vi "4155C Output Config SMUs v2.0.vi"(0 "VISA resource name in":refnum<visa-resource-name>, 1 "sweep method":u16(ring) items=["Continuous", "Pulsed"], 2 "Gate mode":u16(ring)=2 items=["Auto", "Limited", "Fixed"], 3 "Gate Range":u8(slide)=2 max=11 scale=0.0..11.0, 5 "Pulse period":dbl=0.005 min=0.005 max=1.0 step=0.0001 format="%.4f", 7 "Pulse width":dbl=0.0005 min=0.0005 max=0.1 step=0.0001 format="%.4f", 8 "Drain Standby":bool, 9 "Base voltage":dbl format="%^.4e", 10 "Gate Standby":bool, 11 "error in (no error)":errorcluster, 12 "SMU4":cluster{"on/off":bool, "Voltage":dbl} {"Voltage" min=-100.0 max=100.0 format="%.2f"}, 13 "Source/drain mode":u16(ring)=2 items=["Auto", "Limited", "Fixed"], 14 "Source/drain Range":u8(slide)=2 max=11 scale=0.0..11.0) -> (4 "VISA Resource Name out":refnum<visa-resource-name>, 15 "error out":errorcluster)   [LabVIEW 2016]
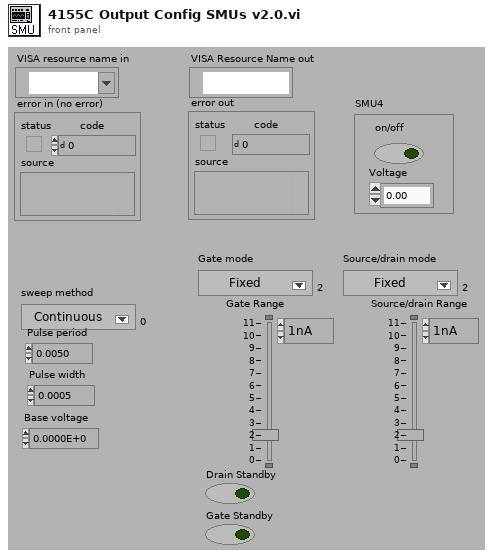
[diagram p1: front panel]
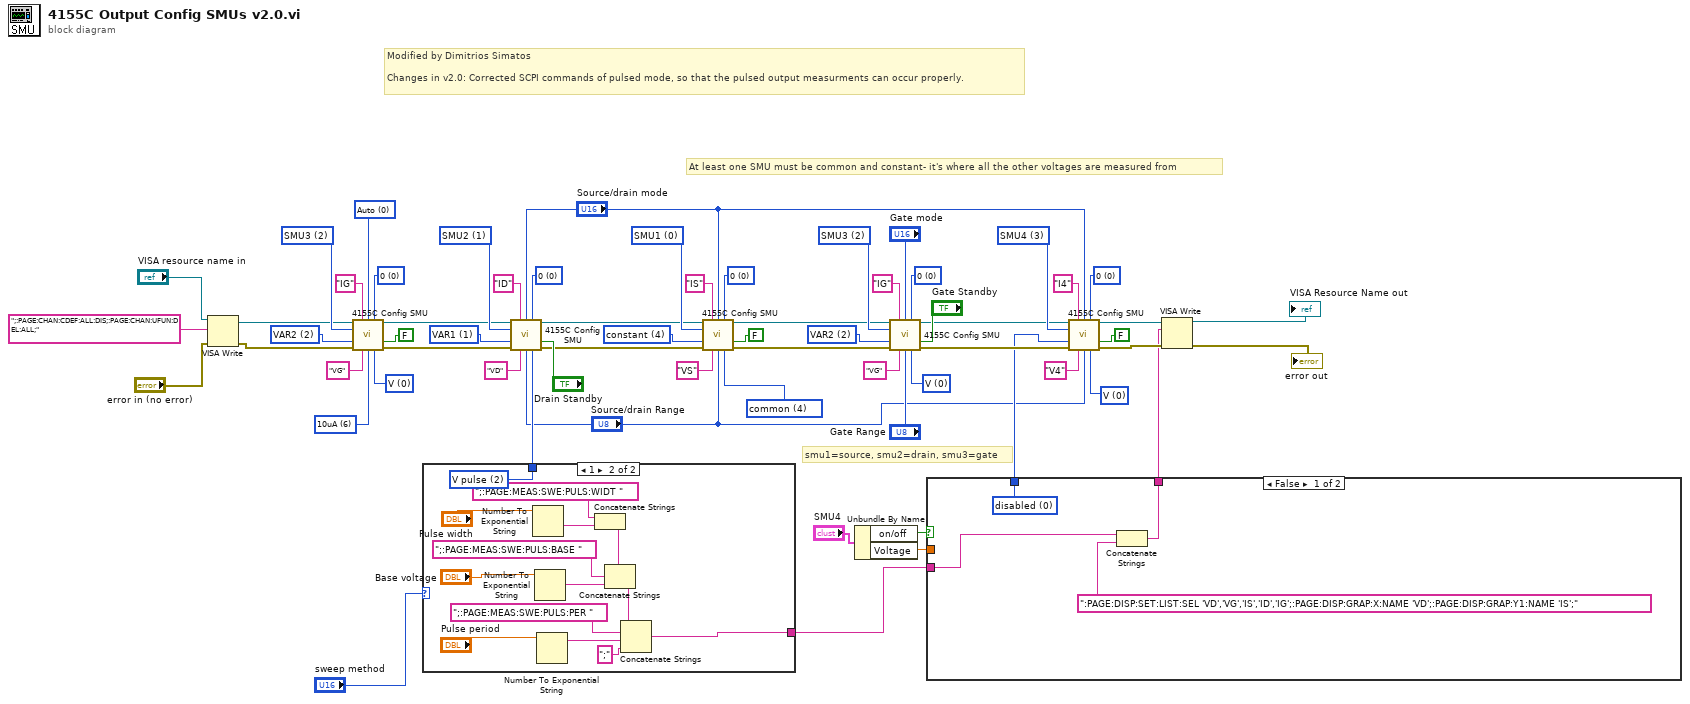
[diagram p0: block diagram]
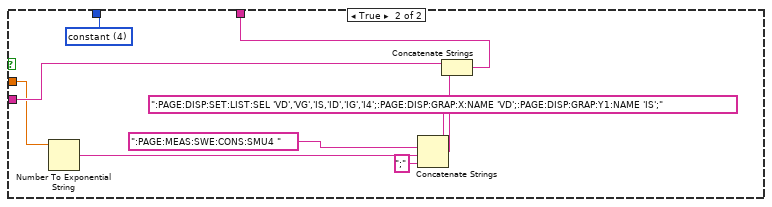
[diagram p2: hidden frame]
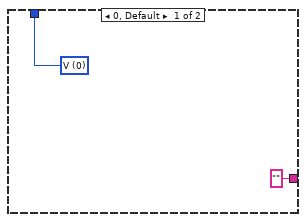
[diagram p3: hidden frame]
diagram:
  w8 = u32 0 items=["V  ", "I  ", "V pulse  ", "I pulse  ", "  common  "] ("mode")
  w15 = u16 0 items=["Auto", "Limited", "Fixed"] ("Range mode")
  w16 = u8 6 items=["10fA  ", "100fA  ", "1nA  ", "10nA", "100nA", "1uA", "10uA", "100uA", "1mA", "10mA", "100mA", "1A"] ("Range")
  w19 = u32 2 items=["SMU1  ", "SMU2  ", "SMU3  ", "SMU4  ", "SMU5  ", "SMU6  "] ("unit to configure")
  w20 = u32 2 items=["disabled  ", "VAR1  ", "VAR2  ", "VAR1'  ", "constant  "] ("function")
  w22 = u32 0 items=["0  ", "10K Ohms  ", "100K Ohms  ", "1M Ohms  "] ("series resistance *")
  w23 = u32 0 items=["V  ", "I  ", "V pulse  ", "I pulse  ", "  common  "] ("mode")
  w43 = u32 0 items=["0  ", "10K Ohms  ", "100K Ohms  ", "1M Ohms  "] ("series resistance *")
  w45 = u32 3 items=["SMU1  ", "SMU2  ", "SMU3  ", "SMU4  ", "SMU5  ", "SMU6  "] ("unit to configure")
  w48 = u32 0 items=["V  ", "I  ", "V pulse  ", "I pulse  ", "  common  "] ("mode")
  w49 = u32 0 items=["0  ", "10K Ohms  ", "100K Ohms  ", "1M Ohms  "] ("series resistance *")
  w51 = u32 2 items=["disabled  ", "VAR1  ", "VAR2  ", "VAR1'  ", "constant  "] ("function")
  w52 = u32 2 items=["SMU1  ", "SMU2  ", "SMU3  ", "SMU4  ", "SMU5  ", "SMU6  "] ("unit to configure")
  w55 = u32 0 items=["0  ", "10K Ohms  ", "100K Ohms  ", "1M Ohms  "] ("series resistance *")
  w57 = u32 4 items=["disabled  ", "VAR1  ", "VAR2  ", "VAR1'  ", "constant  "] ("function")
  w58 = u32 0 items=["SMU1  ", "SMU2  ", "SMU3  ", "SMU4  ", "SMU5  ", "SMU6  "] ("unit to configure")
  w27 = u32 4 items=["V  ", "I  ", "V pulse  ", "I pulse  ", "  common  "] ("mode")
  w61 = u32 0 items=["0  ", "10K Ohms  ", "100K Ohms  ", "1M Ohms  "] ("series resistance *")
  w63 = u32 1 items=["disabled  ", "VAR1  ", "VAR2  ", "VAR1'  ", "constant  "] ("function")
  w64 = u32 1 items=["SMU1  ", "SMU2  ", "SMU3  ", "SMU4  ", "SMU5  ", "SMU6  "] ("unit to configure")
  # "Modified by Dimitrios Simatos\n\nChanges in v2.0: Corrected SCPI commands of pulsed mode, so that the pulsed output measurments can occur properly."
  # "smu1=source, smu2=drain, smu3=gate"
  # "At least one SMU must be common and constant- it's where all the other voltages are measured from"
  n1 = VISA Write(VISA resource name="VISA resource name in", write buffer=";:PAGE:CHAN:CDEF:ALL:DIS;:PAGE:CHAN:UFUN:DEL:ALL;", error in (no error)="error in (no error)") -> (VISA resource name out=w4:refnum<visa-resource-name>, error out=w5:errorcluster)  [unwired: 1 out]
  n2 = call "4155C Config SMU.vi"("VISA session"=w4, "I name (max 6 chars)"="IG", "Range mode"=w15, "series resistance *"=w22, "unit to configure"=w19, "function"=w20, "standby"=FALSE, "error in (no error)"=w5, "V name (max 6 chars)"="VG", "Range"=w16, "mode"=w23) -> ("dup VISA resource name"=w17:refnum<visa-resource-name>, "error out"=w18:errorcluster)  [unwired: 3 in]
  n3 = case shown="1" "sweep method" {
    tunnel: [w66 w80] -> w26
    tunnel: ["" w71] -> w13
    frame 0, Default {
      w66 = u32 0 items=["V  ", "I  ", "V pulse  ", "I pulse  ", "  common  "] ("mode")
    }
    frame 1 {
      w80 = u32 2 items=["V  ", "I  ", "V pulse  ", "I pulse  ", "  common  "] ("mode")
      n4 = Number To Exponential String(number="Pulse width") -> (E-format string=w79:string)  [unwired: 3 in]
      n5 = Number To Exponential String(number="Base voltage") -> (E-format string=w75:string)  [unwired: 3 in]
      n6 = Number To Exponential String(number="Pulse period") -> (E-format string=w72:string)  [unwired: 3 in]
      n7 = Concatenate Strings(";:PAGE:MEAS:SWE:PULS:WIDT " ("Substring"), w79) -> (w77:string)
      n8 = Concatenate Strings(w77, ";:PAGE:MEAS:SWE:PULS:BASE " ("Substring"), w75) -> (w73:string)
      n9 = Concatenate Strings(w73, ";:PAGE:MEAS:SWE:PULS:PER " ("Substring"), w72, ";" ("Substring")) -> (w71:string)
    }
  }
  n10 = call "4155C Config SMU.vi"("VISA session"=w17, "I name (max 6 chars)"="ID", "Range mode"="Source/drain mode", "series resistance *"=w61, "unit to configure"=w64, "function"=w63, "standby"="Drain Standby", "error in (no error)"=w18, "V name (max 6 chars)"="VD", "Range"="Source/drain Range", "mode"=w26) -> ("dup VISA resource name"=w40:refnum<visa-resource-name>, "error out"=w39:errorcluster)  [unwired: 3 in]
  n11 = call "4155C Config SMU.vi"("VISA session"=w40, "I name (max 6 chars)"="IS", "Range mode"="Source/drain mode", "series resistance *"=w55, "unit to configure"=w58, "function"=w57, "standby"=FALSE, "error in (no error)"=w39, "V name (max 6 chars)"="VS", "Range"="Source/drain Range", "mode"=w27) -> ("dup VISA resource name"=w37:refnum<visa-resource-name>, "error out"=w38:errorcluster)  [unwired: 3 in]
  n12 = Unbundle By Name("SMU4") -> ("on/off"=w12:bool, "Voltage"=w10:dbl)
  n13 = call "4155C Config SMU.vi"("VISA session"=w37, "I name (max 6 chars)"="IG", "Range mode"="Gate mode", "series resistance *"=w49, "unit to configure"=w52, "function"=w51, "standby"="Gate Standby", "error in (no error)"=w38, "V name (max 6 chars)"="VG", "Range"="Gate Range", "mode"=w48) -> ("dup VISA resource name"=w36:refnum<visa-resource-name>, "error out"=w35:errorcluster)  [unwired: 3 in]
  n14 = case shown="False" w12 {
    tunnel: w13 -> [w83 w93]
    tunnel: [w82 w92] -> w11
    tunnel: w10 -> [_ w90]
    tunnel: [w81 w91] -> w9
    frame False {
      w81 = u32 0 items=["disabled  ", "VAR1  ", "VAR2  ", "VAR1'  ", "constant  "] ("function")
      n15 = Concatenate Strings(w83, ":PAGE:DISP:SET:LIST:SEL 'VD','VG','IS','ID','IG';:PAGE:DISP:GRAP:X:NAME 'VD';:PAGE:DISP:GRAP:Y1:NAME 'IS';" ("write buffer (\"\")")) -> (w82:string)
    }
    frame True {
      w91 = u32 4 items=["disabled  ", "VAR1  ", "VAR2  ", "VAR1'  ", "constant  "] ("function")
      n16 = Number To Exponential String(number=w90) -> (E-format string=w88:string)  [unwired: 3 in]
      n17 = Concatenate Strings(":PAGE:DISP:SET:LIST:SEL 'VD','VG','IS,'ID','IG','I4';:PAGE:DISP:GRAP:X:NAME 'VD';:PAGE:DISP:GRAP:Y1:NAME 'IS';" ("write buffer (\"\")"), ":PAGE:MEAS:SWE:CONS:SMU4 " ("write buffer (\"\")"), w88, ";" ("Substring")) -> (w86:string)
      n18 = Concatenate Strings(w93, w86) -> (w92:string)
    }
  }
  n19 = call "4155C Config SMU.vi"("VISA session"=w36, "I name (max 6 chars)"="I4", "Range mode"="Source/drain mode", "series resistance *"=w43, "unit to configure"=w45, "function"=w9, "standby"=FALSE, "error in (no error)"=w35, "V name (max 6 chars)"="V4", "Range"="Source/drain Range", "mode"=w8) -> ("dup VISA resource name"=w34:refnum<visa-resource-name>, "error out"=w33:errorcluster)  [unwired: 3 in]
  n20 = VISA Write(VISA resource name=w34, write buffer=w11, error in (no error)=w33) -> (VISA resource name out=→"VISA Resource Name out":refnum<visa-resource-name>, error out=→"error out":errorcluster)  [unwired: 1 out]
